vi "Get Menu Item VI.vi"(7 "Menu Item":string, 8 "error in":errorcluster, 9 "GUID":string, 10 "Item Ref":T1 format="%.0x", 11 "System Explorer Dispatcher in":refnum<class "System Explorer Dispatcher.lvclass">) -> (0 "error out":errorcluster, 2 "menu item reference":refnum<vi>, 3 "System Explorer Dispatcher out":refnum<class "System Explorer Dispatcher.lvclass">)   [LabVIEW 2020, in "AIM MIL-STD-1553 System Explorer.lvlib" / "Implementation.lvlib" / "System Explorer Dispatcher.lvclass"]
uses:
  System Explorer Dispatcher.lvclass
  <vilib>/NI VeriStand/Custom Device API/Custom Device Item Ref.ctl
  Scripting/Constants.vi
  System Explorer/RTM/Export Configuration RTM.vi
  System Explorer/RTM/Import Configuration RTM.vi
  System Explorer/RTM/EnableDisable RTM.vi
  Scripting/AIM MIL-STD-1553 Scripting.lvlib
  Implementation.lvlib
  <vilib>/NI VeriStand/Custom Device API/Custom Device API.lvlib
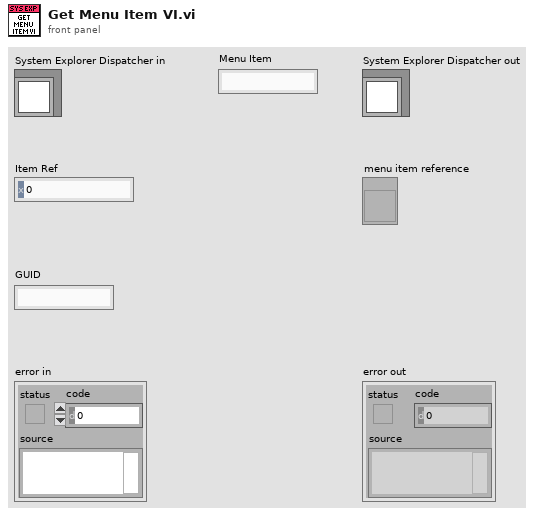
[diagram p1: front panel]
types:
  T1 = typedef "Custom Device API.lvlib/Custom Device Item Ref.ctl" = u64
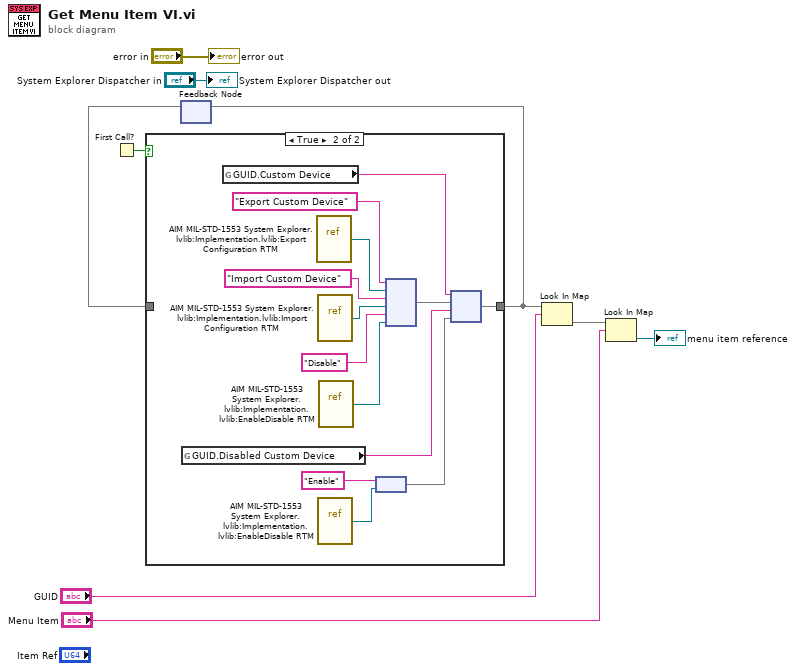
[diagram p0: block diagram]
diagram:
  n1 = First Call?() -> (First Call?: T/F=w7:bool)
  n2 = feedback #1() -> (w2:map{string, map{string, refnum<vi>}})  [unwired: 1 in]
  n3 = case shown="True" w7 {
    tunnel: [w10 w11] -> w3
    tunnel: w2 -> [w10 _]
    frame False {
    }
    frame True {
      n4 = global read "Constants.vi" "GUID.Disabled Custom Device"() -> (w13:string)
      n5 = global read "Constants.vi" "GUID.Custom Device"() -> (w15:string)
      n6 = vi-ref "AIM MIL-STD-1553 System Explorer.lvlib:Implementation.lvlib:Export Configuration RTM.vi"() -> (w22:refnum<vi>)
      n7 = vi-ref "AIM MIL-STD-1553 System Explorer.lvlib:Implementation.lvlib:Import Configuration RTM.vi"() -> (w20:refnum<vi>)
      n8 = vi-ref "AIM MIL-STD-1553 System Explorer.lvlib:Implementation.lvlib:EnableDisable RTM.vi"() -> (w16:refnum<vi>)
      n9 = vi-ref "AIM MIL-STD-1553 System Explorer.lvlib:Implementation.lvlib:EnableDisable RTM.vi"() -> (w18:refnum<vi>)
      n10 = node("Enable" ("Name"), w16) -> (w12:map{string, refnum<vi>})
      n11 = node("Export Custom Device" ("Name"), w22, "Import Custom Device" ("Name"), w20, "Disable" ("Name"), w18) -> (w14:map{string, refnum<vi>})
      n12 = node(w15, w14, w13, w12) -> (w11:map{string, map{string, refnum<vi>}})
    }
  }
  n13 = feedback-in #1(w3) -> ()
  n14 = Look In Map(map=w3, key="GUID") -> (value=w6:map{string, refnum<vi>})  [unwired: 1 in, 1 out]
  n15 = Look In Map(map=w6, key="Menu Item") -> (value=→"menu item reference":refnum<vi>)  [unwired: 1 in, 1 out]
  "error out" <- "error in"
  "System Explorer Dispatcher out" <- "System Explorer Dispatcher in"
